vi "DSF.Shared.Configuration.Framework.From JSON.vi"(8 "error in (no error)":errorcluster, 11 "Framework Configuration in":refnum<class "DSF.Shared.Configuration.Framework.lvclass">) -> (0 "error out":errorcluster, 3 "Framework Configuration out":refnum<class "DSF.Shared.Configuration.Framework.lvclass">)   [LabVIEW 2017, in "DSF.Engine.lvlib" / "DSF.Shared.Configuration.Framework.lvclass"]
uses:
  DSF.Shared.Configuration.Framework.lvclass
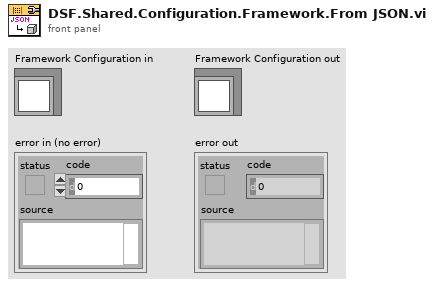
[diagram p1: front panel]
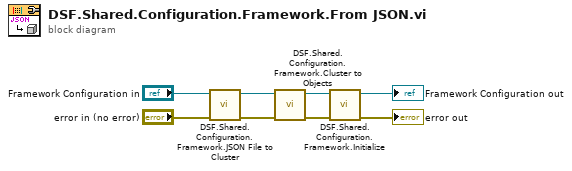
[diagram p0: block diagram]
diagram:
  n1 = call "DSF.Shared.Configuration.Framework.JSON File to Cluster.vi"("error in (no error)"="error in (no error)", "Framework Configuration in"="Framework Configuration in") -> ("error out"=w6:errorcluster, "Framework Configuration out"=w7:refnum<class "DSF.Shared.Configuration.Framework.lvclass">)  [unwired: 8 in]
  n2 = call "DSF.Shared.Configuration.Framework.Cluster to Objects.vi"("error in (no error)"=w6, "Framework Configuration in"=w7) -> ("error out"=w3:errorcluster, "Framework Configuration out"=w4:refnum<class "DSF.Shared.Configuration.Framework.lvclass">)  [unwired: 8 in]
  n3 = call-dynamic "DSF.Shared.Configuration.Framework.Initialize.vi"("error in (no error)"=w3, "Framework Configuration in"=w4) -> ("error out"=→"error out":errorcluster, "Framework Configuration out"=→"Framework Configuration out":refnum<class "DSF.Shared.Configuration.Framework.lvclass">)  [unwired: 8 in]
